vi "Close.vi"(8 "error in (no error)":errorcluster {"code" format="%.0x"}, 11 "instrument handle":refnum<k15>) -> (0 "error out":errorcluster {"code" format="%.0x"})   [LabVIEW 2014, in "Agilent NA.lvlib"]
doc: "Closes the I/O session to the instrument. Driver methods and properties that access the instrument are not accessible after Close is called."
uses:
  Agilent NA.lvlib
  AgNA.dll
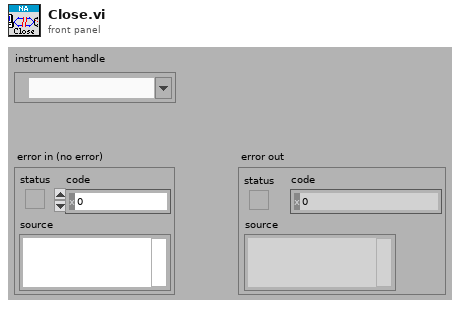
[diagram p1: front panel]
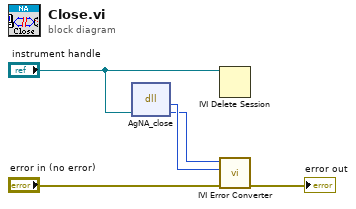
[diagram p0: block diagram]
diagram:
  n1 = dll-call lib="AgNA**.dll" fn="AgNA_close" ("LabVIEW:Ivi_CloseAndGetError")("session"="instrument handle") -> ("return type"=w4:i32, "session"=w3:u32)  [unwired: 3 in, 2 out]
  n2 = IVI Delete Session(11:"instrument handle") -> ()
  n3 = call "IVI Error Converter.vi"("error in (no error)"="error in (no error)", "IVI error code (0)"=w4, "instrument handle"=w3) -> ("error out"=→"error out":errorcluster)  [unwired: 7 in, 1 out]
